vi "FTW-CSV-Variant-Traverse-Cluster.vi"(0 "Variant":variant, 1 "Options":T1={"String Quotes"=FALSE, "Real Format"="%#_15g", "Timestamp Format"="%^<%Y-%m-%dT%H:%M:%S%3uZ>T", "Delimiter"=","}, 11 "error in":errorcluster) -> (4 "CSV String":string, 15 "error out":errorcluster)   [LabVIEW 2015]
uses:
  FTW-CSV-SerializeOptions.ctl
  <vilib>/Utility/Data Type/NI_Data Type.lvlib
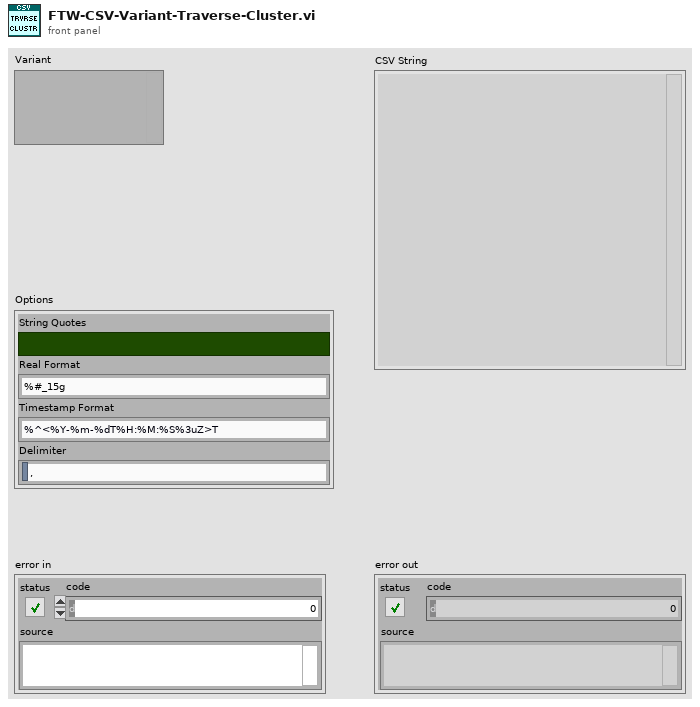
[diagram p1: front panel]
types:
  T1 = typedef "FTW-CSV-SerializeOptions.ctl" = cluster{"String Quotes":bool, "Real Format":string, "Timestamp Format":string, "Delimiter":string}
  T2 = typedef "NI_Data Type.lvlib/Data Type.ctl" = enum8{"Invalid Type", "Void", "I8", "I16", "I32", "I64", "U8", "U16", "U32", "U64", "Single Float", "Double Float", "Extended Float", "Single Complex", "Double Complex", "Extended Complex", "Enum U8", "Enum U16", "Enum U32", "Enum U64", "Single Float With Unit", "Double Float With Unit", "Extended Float With Unit", "Single Complex with Unit", "Double Complex with Unit", "Extended Complex with Unit", "Boolean", "String", "Path", "Picture", "Tag", "Array", "Cluster", "Variant", "LV Variant", "Waveform", "Timestamp", "Digital Waveform", "Digital Data", "ExpressData", "Refnum", "External Data", "VI", "Poly VI", "LabVIEW Class Instance", "Fixed Point"}
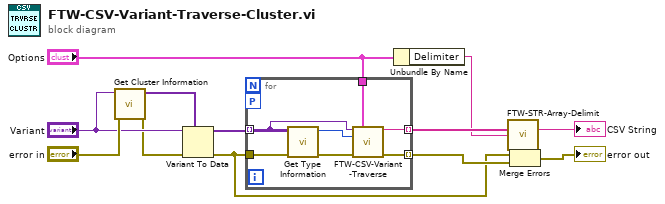
[diagram p0: block diagram]
diagram:
  n1 = call <vilib>:"Get Cluster Information.vi"("error in (no error)"="error in", "Variant"="Variant") -> ("error out"=w5:errorcluster, "Cluster Elements"=w3:variant[])  [unwired: 8 in]
  n2 = Variant To Data(error in=w5, type=w3, Variant="Variant") -> (data=w2:variant[], error out=w4:errorcluster)
  n3 = for {
    tunnel: w2 -> [w14] mode=indexing
    tunnel: [w17] -> w6 mode=indexing
    tunnel: w4 -> [w19]
    tunnel: [w18] -> w7 mode=indexing
    tunnel: "Options" -> [w16]
    workers-P: _ -> [_]
    n4 = call <vilib>:"Get Type Information.vi"("error in (no error)"=w19, "Variant"=w14) -> ("error out"=w15:errorcluster, "Type"=w13:T2)  [unwired: 5 in, 3 out]
    n5 = call "FTW-CSV-Variant-Traverse.vi"("Variant"=w14, "Options"=w16, "Type"=w13, "error in"=w15) -> ("CSV String"=w17:string, "error out"=w18:errorcluster)  [unwired: 10 in]
  }
  n6 = Unbundle By Name("Options") -> ("Delimiter"=w1:string)
  n7 = call "FTW-STR-Array-Delimit.vi"("Array of Strings"=w6, "Delimiter"=w1) -> ("Delimited String"=→"CSV String":string)  [unwired: 13 in]
  n8 = Merge Errors(w4, w7) -> (→"error out":errorcluster)
